vi "Extract Varient.vi"(7 "Copy":bool caption="Copy data instead of extracting", 8 "error in (no error)":errorcluster, 11 "Message":refnum<class "MSG.lvclass">) -> (0 "error out":errorcluster, 1 "Varient":variant, 2 "Label":string, 3 "Message":refnum<class "MSG.lvclass">)   [LabVIEW 2011, in "Messenging.lvlib" / "MSG.lvclass"]
uses:
  MSG.lvclass
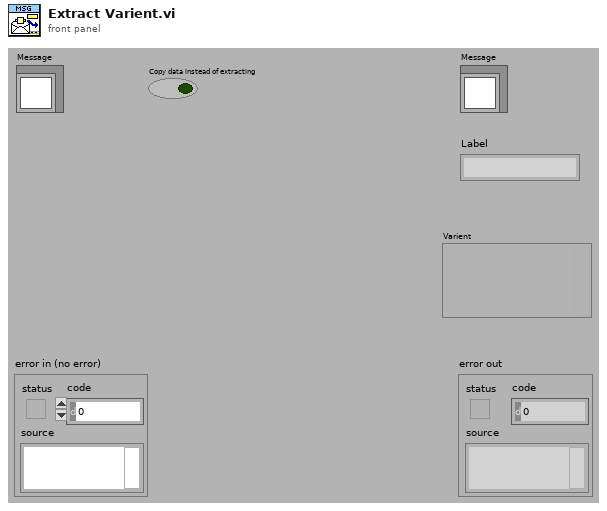
[diagram p1: front panel]
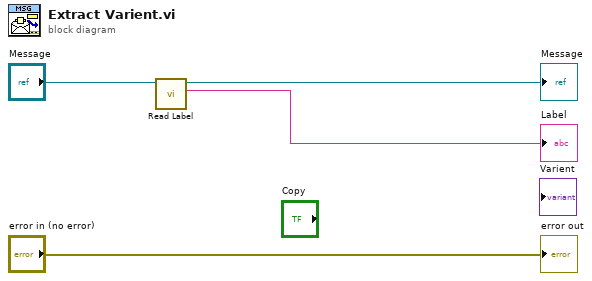
[diagram p0: block diagram]
diagram:
  n1 = call-dynamic "Read Label.vi"("Message"="Message") -> ("Label"=→"Label":string, "Message"=→"Message":refnum<class "MSG.lvclass">)  [unwired: 1 in, 8 out]
  "error out" <- "error in (no error)"
